vi "Wyznaczanie odległości pomiędzy dwoma współrzędnymi geograficznymi.vi"(10 "Współrzędne geograficzne in":string, 11 "Współrzędne geograficzne 1":string) -> (3 "Numeric":dbl)   [LabVIEW 2012, in "Biblioteka moduł map v3.lvlib" / "Matematyczne.lvlib"]
uses:
  Matematyczne.lvlib
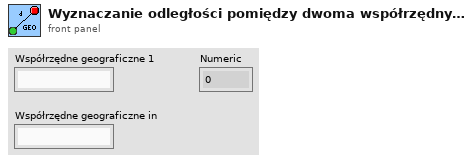
[diagram p1: front panel]
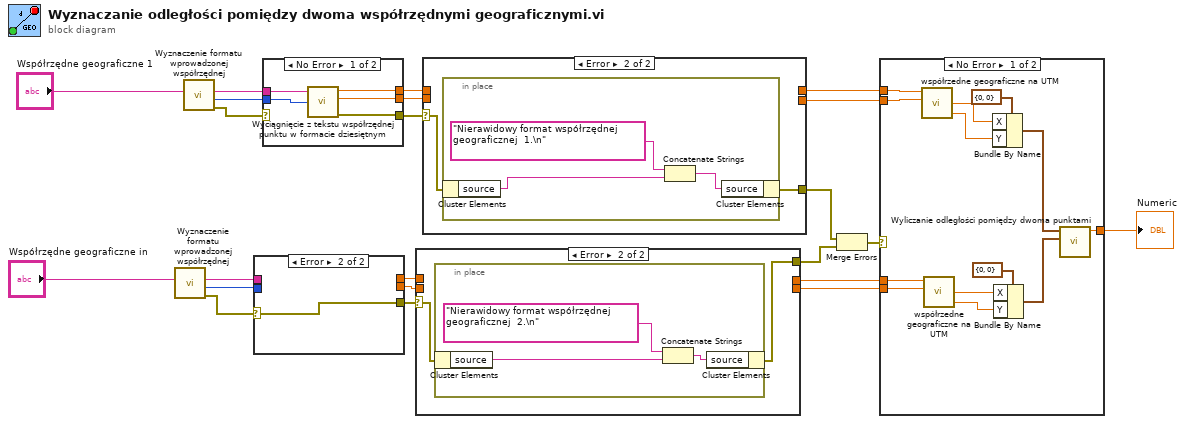
[diagram p0: block diagram]
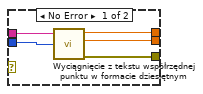
[diagram p3: hidden frame]
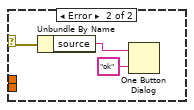
[diagram p4: hidden frame]
diagram:
  n1 = call "Wyznaczenie formatu wprowadzonej współrzędnej.vi"("Współrzędna geograficzna"="Współrzędne geograficzne in") -> ("error constant"=w12:errorcluster, "Format wprowadzonej współrzędnej"=w13:i32, "Znaleziony tekst"=w14:string)  [unwired: 8 in]
  n2 = call "Wyznaczenie formatu wprowadzonej współrzędnej.vi"("Współrzędna geograficzna"="Współrzędne geograficzne 1") -> ("error constant"=w15:errorcluster, "Format wprowadzonej współrzędnej"=w16:i32, "Znaleziony tekst"=w17:string)  [unwired: 8 in]
  n3 = case shown="Error" w12 {
    selector: w12 -> [_ w28]
    tunnel: w14 -> [w27 _]
    tunnel: w13 -> [w26 _]
    tunnel: [w25 _] -> w6
    tunnel: [w24 _] -> w4
    tunnel: [w23 w28] -> w10
    frame No Error {
      n4 = call "Wyciągnięcie z tekstu współrzędnej punktu w formacie dziesiętnym.vi"("Format wprowadzanej współrzędnej"=w26, "Współrzędna w postaci tekstowej"=w27) -> ("error constant"=w23:errorcluster, "Szerokość geograficzna (NS)"=w24:dbl, "Długość geograficzna (EW)"=w25:dbl)  [unwired: 4 in]
    }
    frame Error {
    }
  }
  n5 = case shown="No Error" w15 {
    selector: w15 -> [_ w34]
    tunnel: w17 -> [w33 _]
    tunnel: w16 -> [w32 _]
    tunnel: [w31 _] -> w21
    tunnel: [w30 _] -> w22
    tunnel: [w29 w34] -> w20
    frame No Error {
      n6 = call "Wyciągnięcie z tekstu współrzędnej punktu w formacie dziesiętnym.vi"("Format wprowadzanej współrzędnej"=w32, "Współrzędna w postaci tekstowej"=w33) -> ("error constant"=w29:errorcluster, "Szerokość geograficzna (NS)"=w30:dbl, "Długość geograficzna (EW)"=w31:dbl)  [unwired: 4 in]
    }
    frame Error {
    }
  }
  n7 = case shown="Error" w10 {
    selector: w10 -> [_ w38]
    tunnel: [w36 _] -> w3
    tunnel: w6 -> [w36 _]
    tunnel: [w35 _] -> w5
    tunnel: w4 -> [w35 _]
    tunnel: [_ w37] -> w2
    frame No Error {
    }
    frame Error {
      n8 = in-place {
        n9 = in-place-cluster #1(w38) -> ("source"=w40:string)
        n10 = Concatenate Strings("Nierawidowy format współrzędnej geograficznej  2.\n" ("message"), w40) -> (w39:string)
        n11 = in-place-cluster #1("source"=w39) -> (w37:errorcluster)
      }
    }
  }
  n12 = case shown="Error" w20 {
    selector: w20 -> [_ w45]
    tunnel: w21 -> [w43 _]
    tunnel: w22 -> [w42 _]
    tunnel: [w43 _] -> w8
    tunnel: [w42 _] -> w7
    tunnel: [_ w44] -> w1
    frame No Error {
    }
    frame Error {
      n13 = in-place {
        n14 = in-place-cluster #2(w45) -> ("source"=w47:string)
        n15 = Concatenate Strings("Nierawidowy format współrzędnej geograficznej  1.\n" ("message"), w47) -> (w46:string)
        n16 = in-place-cluster #2("source"=w46) -> (w44:errorcluster)
      }
    }
  }
  n17 = Merge Errors(w1, w2) -> (w9:errorcluster)
  n18 = case shown="No Error" w9 {
    selector: w9 -> [_ w62]
    tunnel: [w53 _] -> w19
    tunnel: w8 -> [w52 _]
    tunnel: w7 -> [w51 _]
    tunnel: w5 -> [w50 _]
    tunnel: w3 -> [w49 _]
    frame No Error {
      n19 = call "współrzedne geograficzne na UTM.vi"("Położenie robota - długość geograficzna"=w52, "Położenie robota - szerokość geograficzna"=w51) -> ("E"=w60:ext, "N"=w59:ext)  [unwired: 4 in, 1 out]
      n20 = call "współrzedne geograficzne na UTM.vi"("Położenie robota - długość geograficzna"=w49, "Położenie robota - szerokość geograficzna"=w50) -> ("E"=w56:ext, "N"=w55:ext)  [unwired: 4 in, 1 out]
      n21 = Bundle By Name(cluster=cluster{"X":i32, "Y":i32} {"X"=0, "Y"=0} ("Polozenie in"), "X"=w60, "Y"=w59) -> (w58:cluster{"X":i32, "Y":i32})
      n22 = Bundle By Name(cluster=cluster{"X":i32, "Y":i32} {"X"=0, "Y"=0} ("Polozenie in"), "X"=w56, "Y"=w55) -> (w54:cluster{"X":i32, "Y":i32})
      n23 = call "Wyliczanie odległości pomiędzy dwoma punktami.vi"("Polozenie 1"=w54, "Polozenie in"=w58) -> ("Numeric"=w53:dbl)  [unwired: 9 in]
    }
    frame Error {
      n24 = Unbundle By Name(w62) -> ("source"=w63:string)
      n25 = One Button Dialog(message=w63, button name ("OK")="ok") -> ()  [unwired: 1 out]
    }
  }
  "Numeric" <- w19
